vi "Set Scaling (None).vi"(8 "error in (no error)":errorcluster, 11 "DAQmx(AI) in":refnum<class "DAQmx(AI).lvclass">) -> (0 "error out":errorcluster, 3 "DAQmx(AI) out":refnum<class "DAQmx(AI).lvclass">)   [LabVIEW 2013, in "DAQmx(AI).lvclass"]
uses:
  DAQmx(AI).lvclass
  Typedefs/ScalingType--Enum.ctl
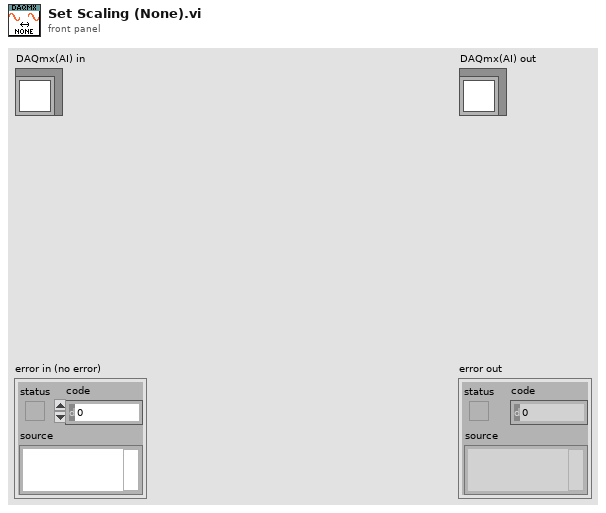
[diagram p1: front panel]
types:
  T1 = typedef "DAQmx(AI).lvclass/ScalingType--Enum.ctl" = enum16{"No scaling", "Linear", "Map Range", "Polynomial", "Table"}
  T2 = typedef "DAQmx(AI).lvclass/Scaling--Cluster.ctl" = cluster{"Scale Name":string, "Scale Type":T1, "Scaled Units":string, "Linear":T3, "Map Range":T4, "Polynomial":T5, "Table":T6}
  T3 = typedef "DAQmx(AI).lvclass/Scaling(Linear)--Cluster.ctl" = cluster{"Slope":dbl, "Intercept":dbl}
  T4 = typedef "DAQmx(AI).lvclass/Scaling(MapRange)--Cluster.ctl" = cluster{"Minimum":dbl, "Maximum":dbl}
  T5 = typedef "DAQmx(AI).lvclass/Scaling(Polynomial)--Cluster.ctl" = cluster{"forward coeff":dbl[], "reverse coeff":dbl[]}
  T6 = typedef "DAQmx(AI).lvclass/Scaling(Table)--Cluster.ctl" = cluster{"scaled values":dbl[], "pres-scaled values":dbl[]}
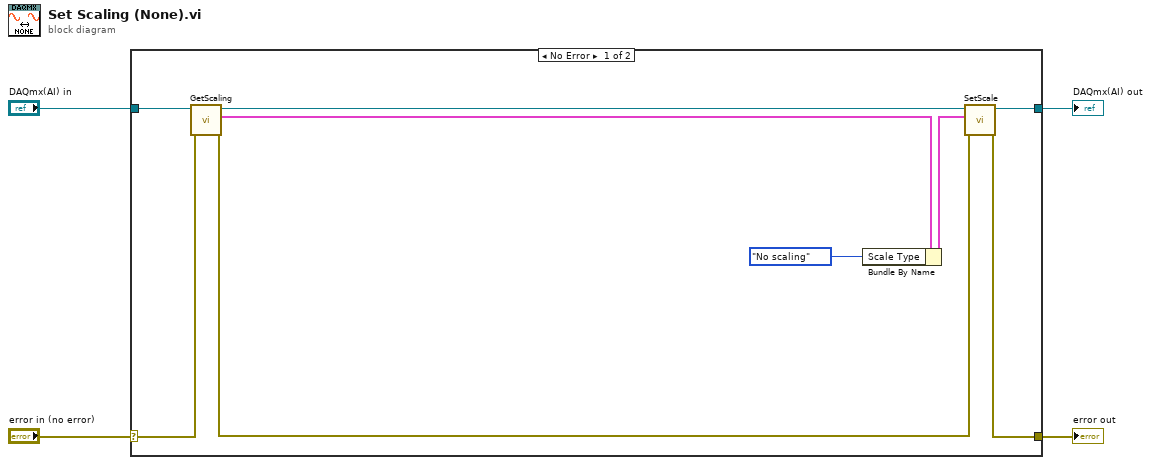
[diagram p0: block diagram]
diagram:
  n1 = case shown="No Error" "error in (no error)" {
    selector: "error in (no error)" -> [w9 w15]
    tunnel: [w12 w15] -> w3
    tunnel: [w13 w14] -> w1
    tunnel: "DAQmx(AI) in" -> [w11 w14]
    frame No Error {
      n2 = call "GetScaling.vi"("error in (no error)"=w9, "Subsystem"=w11) -> ("error out"=w6:errorcluster, "Scaling"=w5:T2, "Subsystem out"=w10:refnum<class "DAQmx(AI).lvclass">)  [unwired: 6 in, 1 out]
      n3 = Bundle By Name(cluster=w5, "Scale Type"=ScalingType--Enum."No scaling") -> (w7:T2)
      n4 = call "SetScale.vi"("error in (no error)"=w6, "Scaling"=w7, "Subsystem"=w10) -> ("error out"=w12:errorcluster, "Subsystem out"=w13:refnum<class "DAQmx(AI).lvclass">)  [unwired: 7 in]
    }
    frame Error {
    }
  }
  "error out" <- w3
  "DAQmx(AI) out" <- w1
